vi "Scan_ver2.vi"(0 "DMM ref":refnum<visa-resource-name>, 1 "output cluster":cluster{"Timeout":i32, "Channel number":i32}, 2 "P_current_count":i32, 3 "N_current_count":i32, 5 "DMM error":errorcluster, 7 "Current Sense \nResitance Array":dbl[](array[numeric])=[1.0032214, 1.00250644, 1.00234822, 1.0040944, 1.0017711, 1.00229431, 1.00344206, 1.00482066, 1.00381056, 1.00290978, 1.00333016, 1.00367587], 9 "ESP32 ref":refnum<visa-resource-name>, 11 "ESP32 error":errorcluster, 12 "current_mode":u8[](array[numeric])=[0, 0, 0, 0, 0, 0, 0, 0, 0, 0, 0]) -> (4 "DMM ref":refnum<visa-resource-name>, 6 "DMM error":errorcluster, 8 "Measurements":dbl[](array[numeric]), 10 "ESP32 ref":refnum<visa-resource-name>, 13 "Timout?":bool, 14 "Time out count":i32, 15 "ESP32 error":errorcluster)   [LabVIEW 2023]
uses:
  <instrlib>/Agilent 3446X Series/Agilent 3446X Series.lvlib
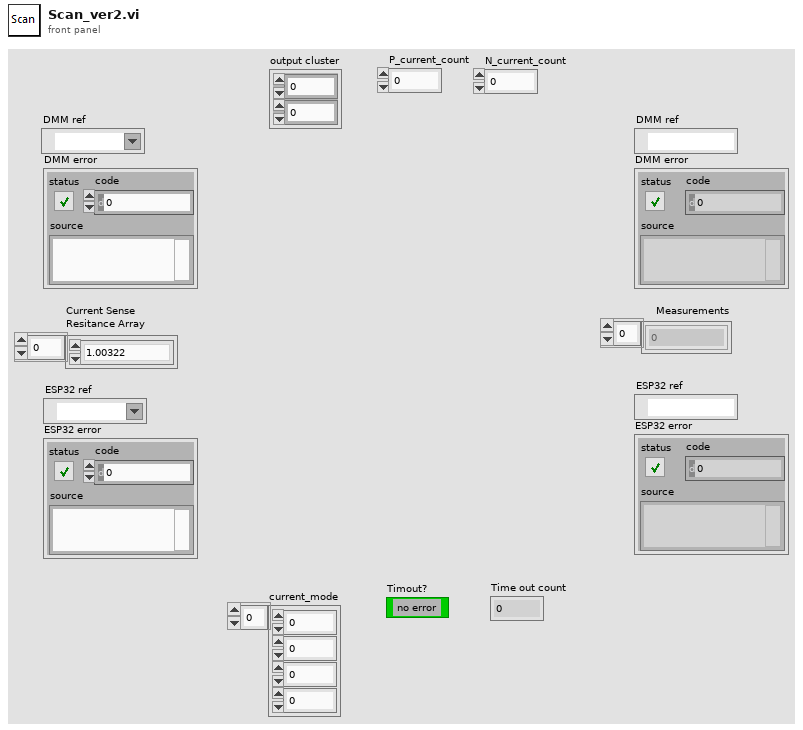
[diagram p1: front panel]
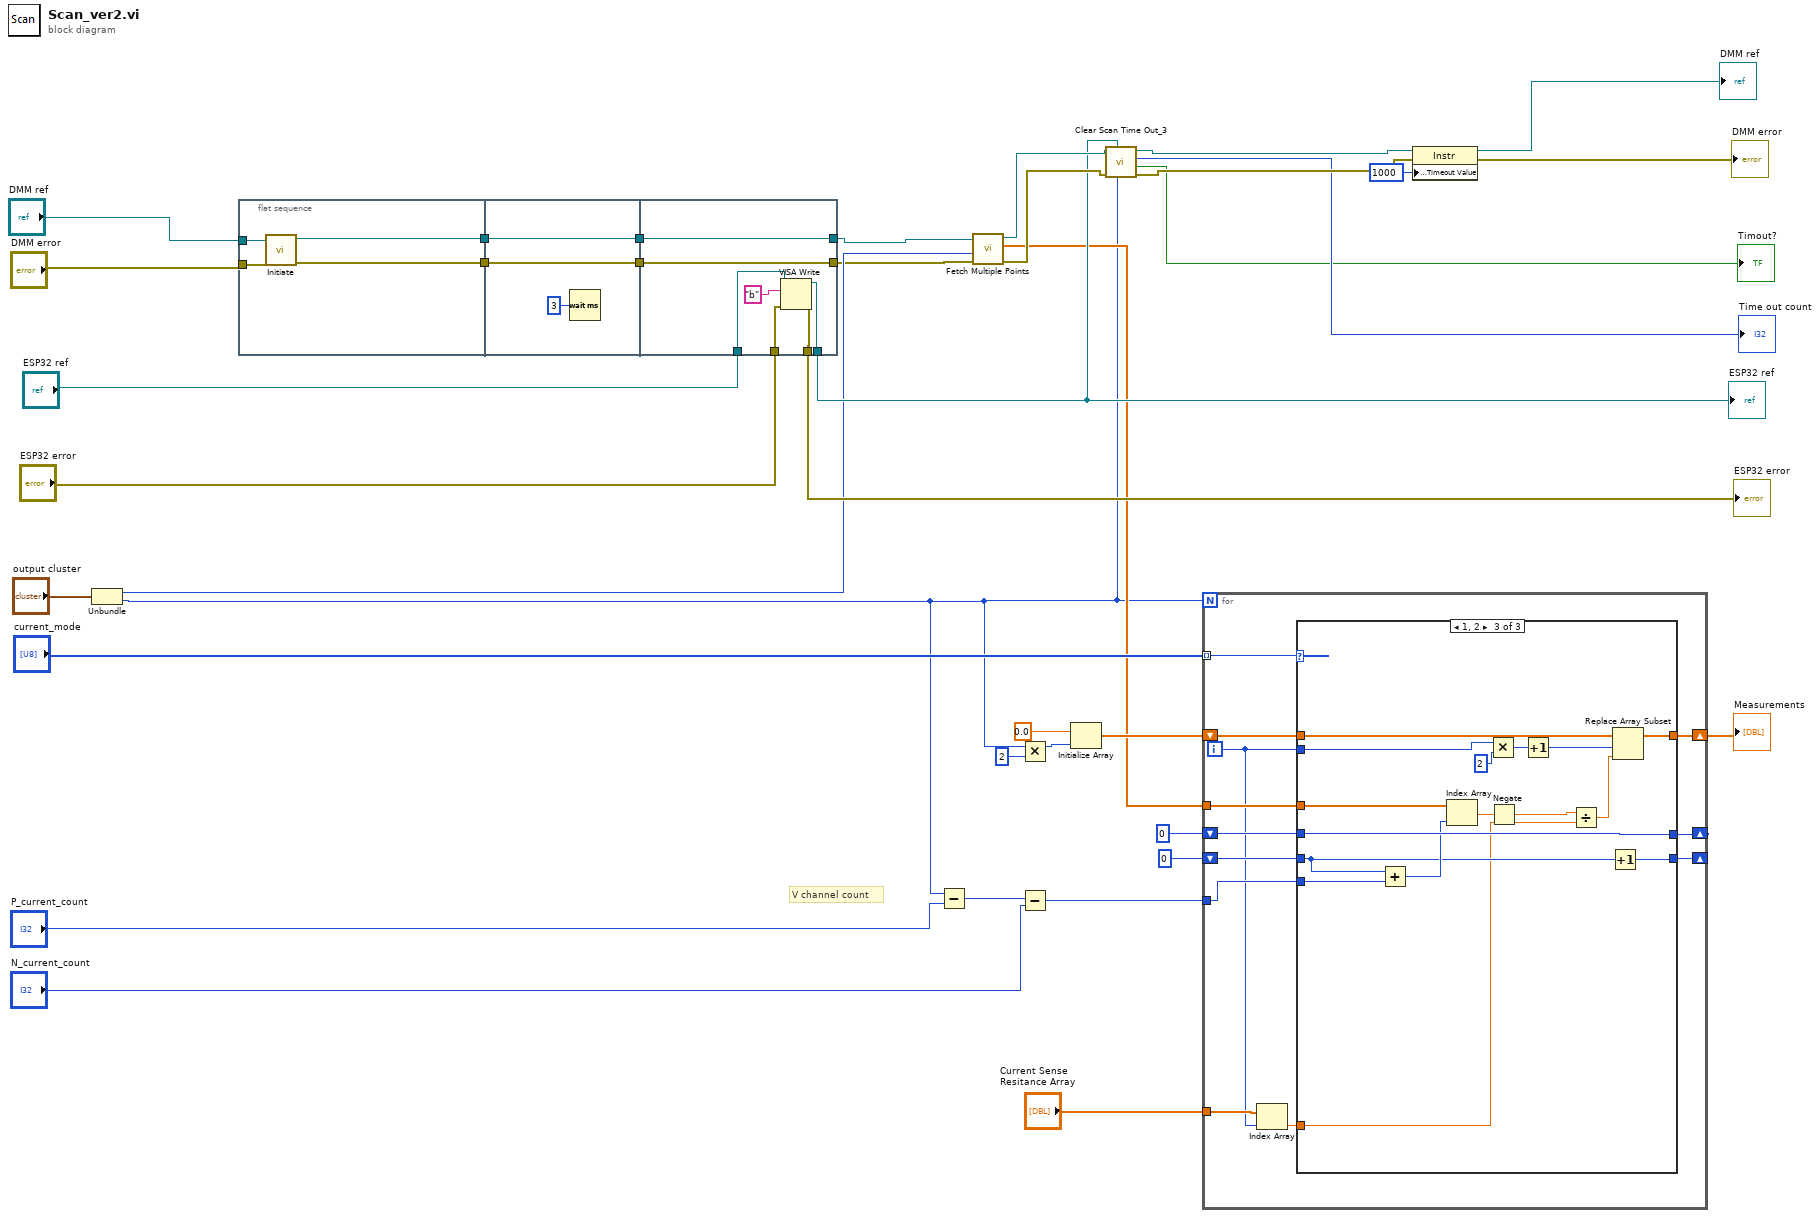
[diagram p0: block diagram]
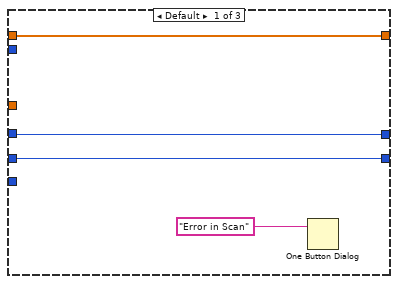
[diagram p2: hidden frame]
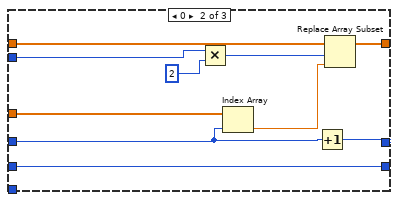
[diagram p3: hidden frame]
diagram:
  # "V channel count"
  n1 = Unbundle("output cluster") -> ("Timeout"=w4:i32, "Channel number"=w1:i32)
  n2 = flat-sequence {
    tunnel: [w42] -> w38
    tunnel: [w41] -> w37
    tunnel: "DMM ref" -> [w40]
    tunnel: "DMM error" -> [w39]
    tunnel: w38 -> [w45]
    tunnel: [w45] -> w36
    tunnel: w37 -> [w44]
    tunnel: [w44] -> w35
    tunnel: w36 -> [w52]
    tunnel: w35 -> [w51]
    tunnel: "ESP32 ref" -> [w50]
    tunnel: "ESP32 error" -> [w49]
    tunnel: [w48] -> w24
    tunnel: [w47] -> w25
    tunnel: [w52] -> w3
    tunnel: [w51] -> w2
    frame #0 {
      n3 = call <instrlib>:"Initiate.vi"("error in (no error)"=w39, "VISA resource name"=w40) -> ("error out"=w42:errorcluster, "VISA resource name out"=w41:refnum<visa-resource-name>)  [unwired: 8 in]
    }
    frame #1 {
      n4 = Wait (ms)(milliseconds to wait=u32 3) -> ()  [unwired: 1 out]
    }
    frame #2 {
      n5 = VISA Write(VISA resource name=w50, write buffer="b" ("data in"), error in (no error)=w49) -> (VISA resource name out=w48:refnum<visa-resource-name>, error out=w47:errorcluster)  [unwired: 1 out]
    }
  }
  n6 = Subtract(x=w1, y="P_current_count") -> (x-y=w15:i32)
  n7 = call <instrlib>:"Fetch Multiple Points.vi"("error in (no error)"=w3, "Timeout (10000 ms)"=w4, "VISA resource name"=w2) -> ("error out"=w32:errorcluster, "Measurements"=w16:dbl[], "VISA resource name out"=w33:refnum<visa-resource-name>)  [unwired: 1 in, 5 out]
  n8 = Multiply(x=w1, y=2) -> (x*y=w20:i32)
  n9 = Subtract(x=w15, y="N_current_count") -> (x-y=w14:i32)
  n10 = Initialize Array(0.0 ("Measurement"), w20) -> (w18:dbl[])
  n11 = call "Clear Scan Time Out_3.vi"("Channel number"=w1, "ESP32 ref"=w24, "error in (no error)"=w32, "VISA Refnum in"=w33) -> ("error out"=w30:errorcluster, "error?"=→"Timout?":bool, "Time out count"=→"Time out count":i32, "VISA Refnum out"=w31:refnum<visa-resource-name>)  [unwired: 3 in, 1 out]
  n12 = for {
    N: w1 -> [_]
    shift-right: [w59] -> w9
    shift-left: w18 -> [w60]
    tunnel: "current_mode" -> [w64] mode=indexing
    tunnel: w16 -> [w63]
    tunnel: w14 -> [w56]
    shift-right: [w61] -> _
    shift-left: 0 ("index") -> [w62]
    shift-right: [w57] -> _
    shift-left: 0 ("index") -> [w58]
    tunnel: "Current Sense \nResitance Array" -> [w55]
    i -> [w54]
    n13 = Index Array(array=w55, index=w54) -> (element=w53:dbl)
    n14 = case shown="1, 2" w64 {
      tunnel: w63 -> [_ w78 w87]
      tunnel: w62 -> [w68 w76 w88]
      tunnel: [w68 w75 w88] -> w61
      tunnel: w54 -> [_ w73 w93]
      tunnel: w60 -> [w67 w74 w94]
      tunnel: [w67 w71 w90] -> w59
      tunnel: w58 -> [w66 w70 w84]
      tunnel: [w66 w70 w83] -> w57
      tunnel: w56 -> [_ _ w86]
      tunnel: w53 -> [_ _ w80]
      frame Default {
        n15 = One Button Dialog(message="Error in Scan") -> ()  [unwired: 1 in, 1 out]
      }
      frame 0 {
        n16 = Multiply(x=w73, y=2 ("x")) -> (x*y=w69:i32)
        n17 = Index Array(array=w78, index=w76) -> (element=w77:dbl)
        n18 = Increment(x=w76) -> (x+1=w75:i32)
        n19 = Replace Array Subset(array=w74, new element=w77, index=w69) -> (w71:dbl[])
      }
      frame 1, 2 {
        n20 = Add(x=w84, y=w86) -> (x+y=w85:i32)
        n21 = Index Array(array=w87, index=w85) -> (element=w81:dbl)
        n22 = Multiply(x=w93, y=2 ("x")) -> (x*y=w91:i32)
        n23 = Negate(x=w81) -> (-x=w79:dbl)
        n24 = Increment(x=w91) -> (x+1=w89:i32)
        n25 = Divide(x=w79, y=w80) -> (x/y=w82:dbl)
        n26 = Increment(x=w84) -> (x+1=w83:i32)
        n27 = Replace Array Subset(array=w94, new element=w82, index=w89) -> (w90:dbl[])
      }
    }
  }
  "Measurements" <- w9
  n28 = property class="Instr"(reference=w31, error in=w30, "General Settings:Timeout Value"=u32 1000) -> (reference out=→"DMM ref":refnum<visa-resource-name>, error out=→"DMM error":errorcluster)
  "ESP32 ref" <- w24
  "ESP32 error" <- w25
